vi "Write Element of Opened SMOs.vi"(8 "error in (no error)":errorcluster, 9 "SMO.lvclass":refnum<class "SMO.lvclass">, 10 "index":i32, 11 "Test.Maui 2.0.Panels in":refnum<class "Test.Maui 2.0.Panels.lvclass">) -> (0 "error out":errorcluster, 3 "Test.Maui 2.0.Panels out":refnum<class "Test.Maui 2.0.Panels.lvclass">)   [LabVIEW 2020, in "Test.Maui 2.0.Panels.lvclass"]
uses:
  Test.Maui 2.0.Panels.lvclass
  <vilib>/JKI/JKI SMO/SMO/SMO.lvclass
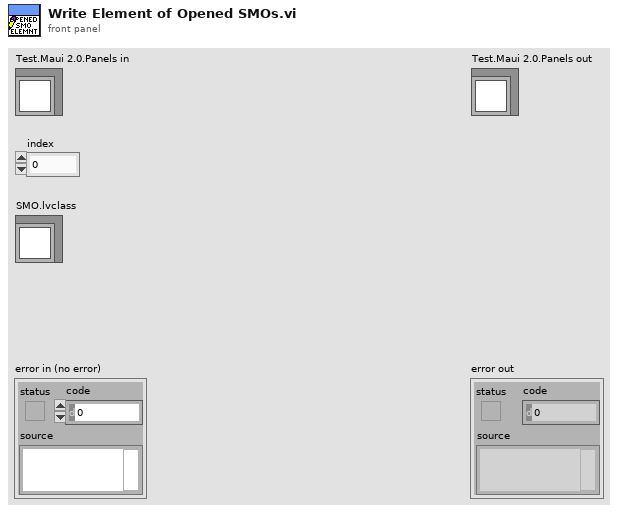
[diagram p1: front panel]
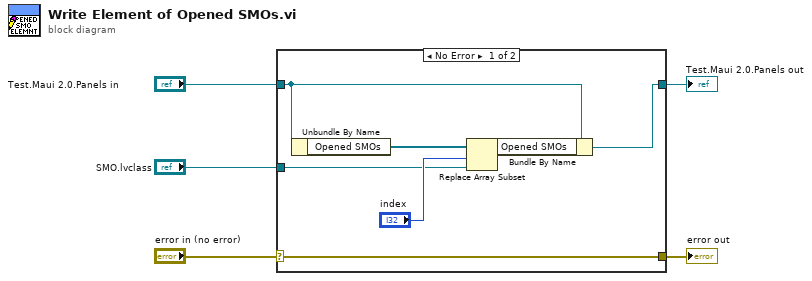
[diagram p0: block diagram]
diagram:
  n1 = case shown="No Error" "error in (no error)" {
    selector: "error in (no error)" -> [w12 w13]
    tunnel: [w12 w13] -> w4
    tunnel: [w11 w14] -> w2
    tunnel: "Test.Maui 2.0.Panels in" -> [w10 w14]
    tunnel: "SMO.lvclass" -> [w6 _]
    frame No Error {
      n2 = Unbundle By Name(w10) -> ("Opened SMOs"=w9:refnum<class "SMO.lvclass">[])
      n3 = Replace Array Subset(array=w9, new element=w6, index="index") -> (w8:refnum<class "SMO.lvclass">[])
      n4 = Bundle By Name(cluster=w10, "Opened SMOs"=w8) -> (w11:refnum<class "Test.Maui 2.0.Panels.lvclass">)
    }
    frame Error {
    }
  }
  "error out" <- w4
  "Test.Maui 2.0.Panels out" <- w2
